vi "Progress Bar State.vi"(8 "error in (no error)":errorcluster, 9 "String In":string, 10 "Progress In":u8, 11 "Progress Actions":T1) -> (0 "error out":errorcluster, 1 "String Out":string, 2 "Exit Out":bool, 3 "Progress Out":u8)   [LabVIEW 2013]
uses:
  Progress Bar Actions.ctl
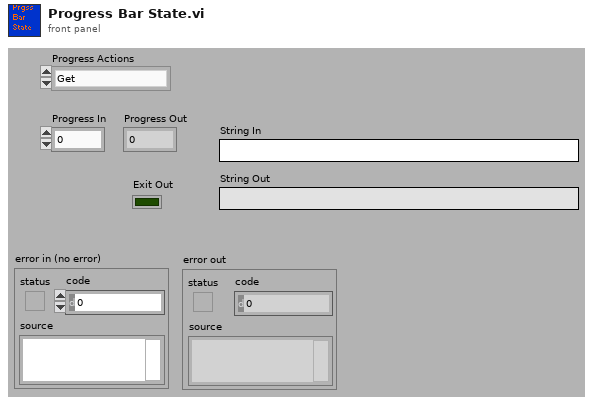
[diagram p1: front panel]
types:
  T1 = typedef "Progress Bar Actions.ctl" = enum16{"Get", "Set", "Exit", "Init"}
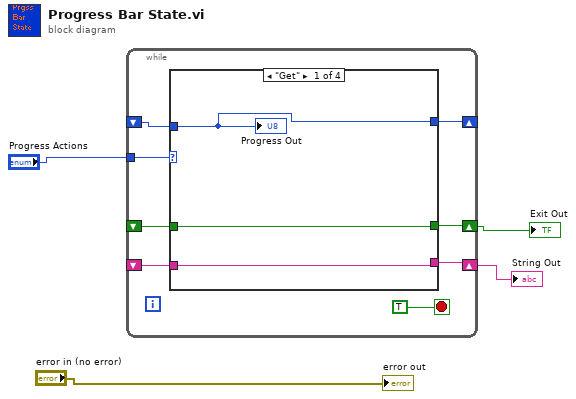
[diagram p0: block diagram]
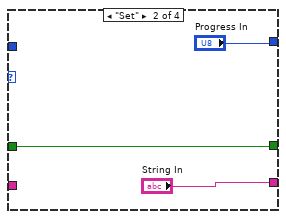
[diagram p2: hidden frame]
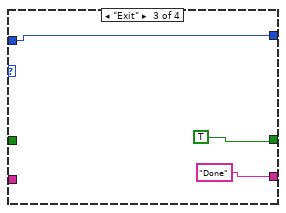
[diagram p3: hidden frame]
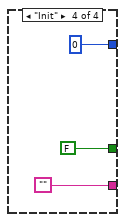
[diagram p4: hidden frame]
diagram:
  n1 = while {
    tunnel: "Progress Actions" -> [w11]
    shift-right: [w10] -> _
    shift-left: _ -> [w8]
    shift-right: [w9] -> w3
    shift-left: _ -> [w7]
    shift-right: [w6] -> w1
    shift-left: _ -> [w5]
    stop <- TRUE stop-if-true
    n2 = case shown="\"Get\"" w11 {
      tunnel: [w15 "Progress In" w21 u8 0 ("Progress Out")] -> w10
      tunnel: [w14 w17 TRUE FALSE] -> w9
      tunnel: w8 -> [w15 _ w21 _]
      tunnel: w7 -> [w14 w17 _ _]
      tunnel: [w13 "String In" "Done" ""] -> w6
      tunnel: w5 -> [w13 _ _ _]
      frame "Get" {
        "Progress Out" <- w15
      }
      frame "Set" {
      }
      frame "Exit" {
      }
      frame "Init" {
      }
    }
  }
  "Exit Out" <- w3
  "String Out" <- w1
  "error out" <- "error in (no error)"
